vi "error message1.vi"() -> (2 "Next action":bool)   [LabVIEW 2015]
panel:
  in  "No":bool
  in  "Yes":bool
  out "Boolean":bool
  out "Message":string
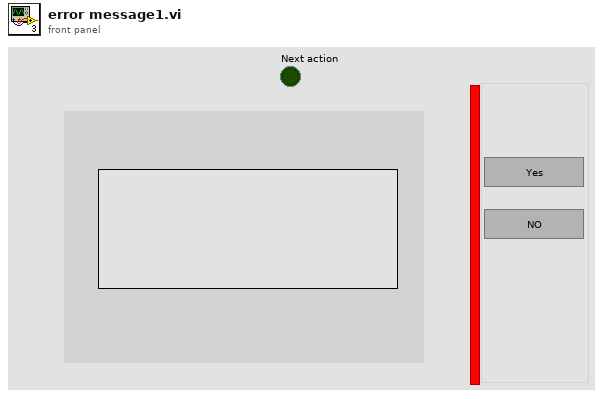
[diagram p1: front panel]
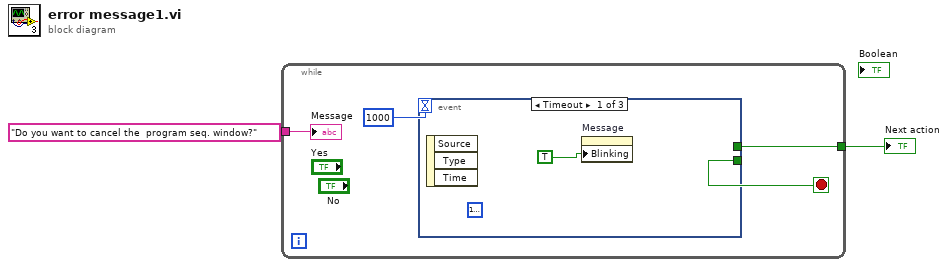
[diagram p0: block diagram]
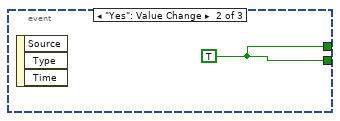
[diagram p2: hidden frame]
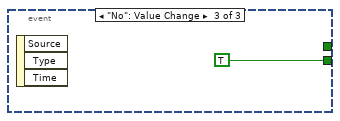
[diagram p3: hidden frame]
diagram:
  n1 = while {
    tunnel: [w5] -> w2
    tunnel: "Do you want to cancel the  program seq. window?" ("Message") -> [w4]
    stop <- w6 stop-if-true
    n2 = event shown="[0] Timeout" {
      selector: _ -> [_ _ _]
      dyn-events: _ -> [_ _ _]
      timeout: 1000 -> [_ _ _]
      tunnel: [_ w8 TRUE] -> w6
      tunnel: [_ w8 _] -> w5
      event Timeout {
        (unwired) u32 16777225 ("Color Box")
        n3 = event-data() -> ()  [unwired: 1 in, 3 out]
        n4 = property on="Message" class="Str"("Blinking"=TRUE) -> ()  [unwired: 2 in, 2 out]
      }
      event "Yes": Value Change {
        w8 = TRUE
        n5 = event-data() -> ()  [unwired: 1 in, 3 out]
      }
      event "No": Value Change {
        n6 = event-data() -> ()  [unwired: 1 in, 3 out]
      }
    }
    "Message" <- w4
  }
  "Next action" <- w2
